vi "Power (1 Channel).vi"(8 "error in (no error)":errorcluster, 10 "current waveform":waveform(dbl), 11 "voltage waveform":waveform(dbl)) -> (0 "error out":errorcluster, 3 "power value":T1)   [LabVIEW 2013, in "NI_EP_Basic.lvlib"]
doc: "Calculates the power values from a voltage and current signal. Wire data to the <B>voltage waveform</B> input or the <B>current waveform</B> input to determine the polymorphic instance to use or manually select the instance."
uses:
  <vilib>/addons/Electrical Power/Basic/NI_EP_Basic.lvlib
  <vilib>/addons/Electrical Power/Basic/Measurement/subVIs/basic_Power Value.ctl
  <vilib>/Analysis/baseanly.llb/Mean (DBL).vi
  <vilib>/addons/Electrical Power/Basic/Measurement/RMS (1 Channel).vi
  <vilib>/Analysis/NI_AALBase.lvlib
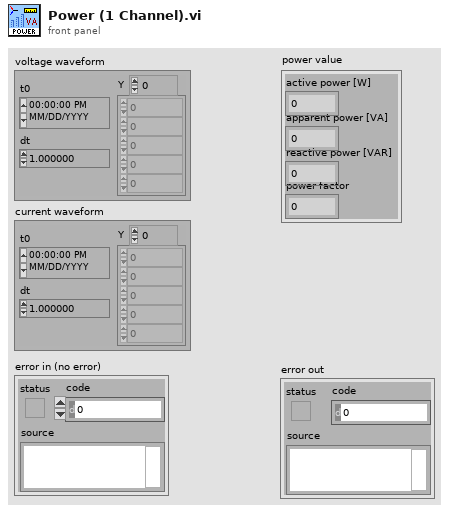
[diagram p1: front panel]
types:
  T1 = typedef "NI_EP_Basic.lvlib/basic_Power Value.ctl" = cluster{"active power [W]":dbl, "apparent power [VA]":dbl, "reactive power [VAR]":dbl, "power factor":dbl}
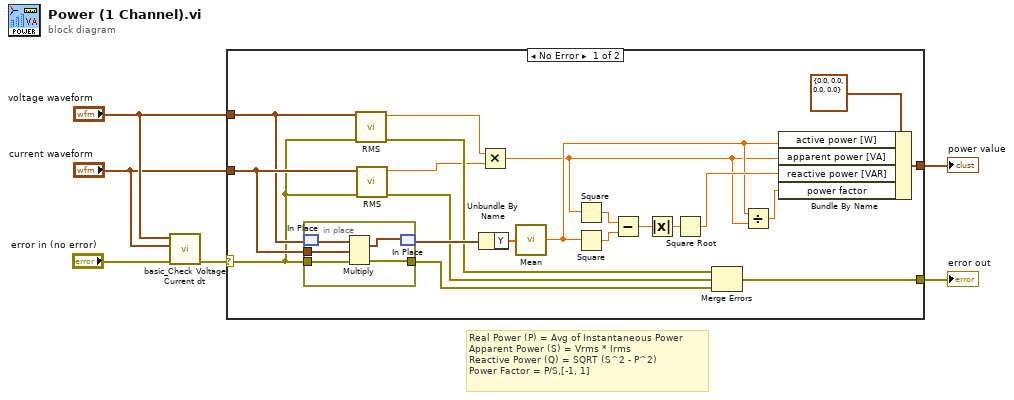
[diagram p0: block diagram]
diagram:
  # "Real Power (P) = Avg of Instantaneous Power\nApparent Power (S) = Vrms * Irms\nReactive Power (Q) = SQRT (S^2 - P^2)\nPower Factor = P/S,[-1, 1]"
  n1 = call <vilib>:"basic_Check Voltage Current dt.vi"("error in (no error)"="error in (no error)", "current waveform"="current waveform", "voltage waveform"="voltage waveform") -> ("error out"=w3:errorcluster)  [unwired: 8 in]
  n2 = case shown="No Error" w3 {
    selector: w3 -> [w15 w33]
    tunnel: [w11 w33] -> w6
    tunnel: "current waveform" -> [w17 _]
    tunnel: "voltage waveform" -> [w16 _]
    tunnel: [w21 _] -> w5
    frame No Error {
      n3 = in-place {
        in-place-border: w17 -> [w32]
        in-place-border: w15 -> [w29]
        in-place-border: [w28] -> w12
        n4 = in-place-match #1(w16) -> (w31:waveform(dbl))
        n5 = Multiply(1:w32, 2:w31, 4:w29) -> (0:w30:waveform(dbl), 3:w28:errorcluster)
        n6 = in-place-match #1(w30) -> (w19:waveform(dbl))
      }
      n7 = call-poly <vilib>:"RMS.vi"("error in (no error)"=w15, "waveform"=w16) -> ("error out"=w14:errorcluster, "RMS value"=w10:dbl)  [unwired: 8 in]
      n8 = call-poly <vilib>:"RMS.vi"("error in (no error)"=w15, "waveform"=w17) -> ("error out"=w13:errorcluster, "RMS value"=w9:dbl)  [unwired: 8 in]
      n9 = Unbundle By Name(w19) -> ("Y"=w18:dbl[])
      n10 = Multiply(x=w10, y=w9) -> (x*y=w7:dbl)
      n11 = call-poly <vilib>:"Mean.vi"("X"=w18) -> ("mean"=w20:dbl)  [unwired: 1 out]
      n12 = Square(x=w7) -> (x^2=w26:dbl)
      n13 = Square(x=w20) -> (x^2=w27:dbl)
      n14 = Subtract(x=w26, y=w27) -> (x-y=w25:dbl)
      n15 = Absolute Value(x=w25) -> (abs(x)=w24:dbl)
      n16 = Square Root(x=w24) -> (sqrt(x)=w22:dbl)
      n17 = Merge Errors(w14, w13, w12) -> (w11:errorcluster)
      n18 = Divide(x=w20, y=w7) -> (x/y=w23:dbl)
      n19 = Bundle By Name(cluster=T1 {"active power [W]"=0.0, "apparent power [VA]"=0.0, "reactive power [VAR]"=0.0, "power factor"=0.0} ("power value"), "active power [W]"=w20, "apparent power [VA]"=w7, "reactive power [VAR]"=w22, "power factor"=w23) -> (w21:T1)
    }
    frame Error {
    }
  }
  "error out" <- w6
  "power value" <- w5
